vi "Write ITX (1D).vi"(0 "Commands":string, 5 "filename":path, 7 "Notes":string, 8 "Array name":string, 9 "1D Array":dbl[](array[numeric])) -> ()   [LabVIEW 2016, in "Data.ITX.lvclass"]
uses:
  Data.ITX.lvclass
  Data/Data.lvclass
panel:
  out "String":string
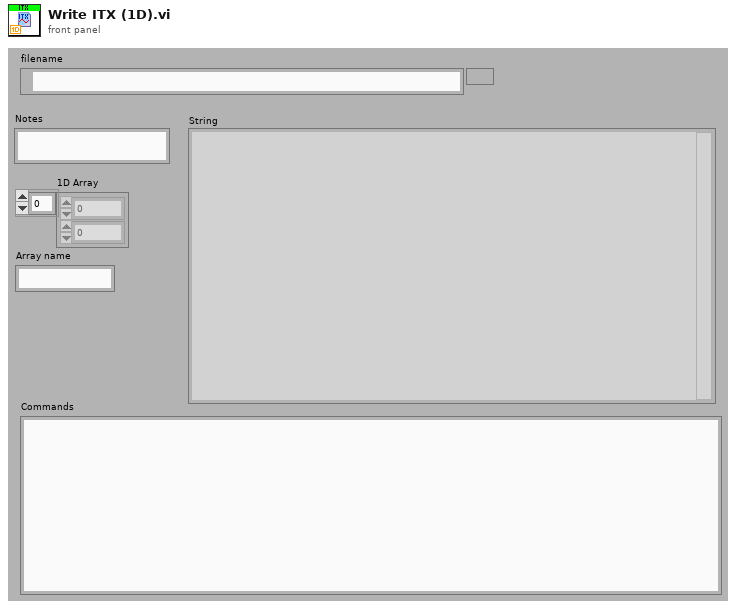
[diagram p1: front panel]
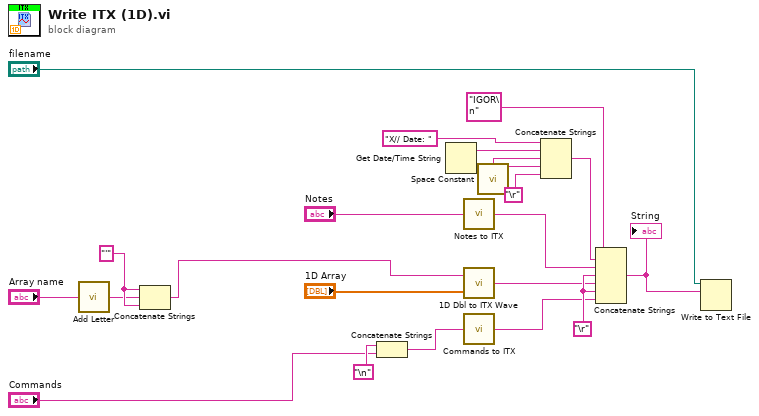
[diagram p0: block diagram]
diagram:
  w3 = "'" ("string")
  w17 = "\r"
  n1 = call "Add Letter.vi"("String"="Array name") -> ("output string"=w2:string)
  n2 = Concatenate Strings(w3, w2, w3) -> (w1:string)
  n3 = Concatenate Strings("\n", "Commands") -> (w8:string)
  n4 = Get Date/Time String() -> (date string=w21:string, time string=w22:string)  [unwired: 3 in]
  n5 = call "Notes to ITX.vi"("Notes"="Notes") -> ("ITX Notes"=w9:string)
  n6 = call "1D Dbl to ITX Wave.vi"("1D Array"="1D Array", "Wavename"=w1) -> ("ITX Wave"=w5:string)
  n7 = call "Commands to ITX.vi"("Commands"=w8) -> ("ITX Commands"=w7:string)
  n8 = call <vilib>:"Space Constant.vi"() -> ("String"=w15:string)
  n9 = Concatenate Strings("X// Date: " ("format string"), w21, w15, w22, "\r") -> (w20:string)
  n10 = Concatenate Strings("IGOR\n", w20, w9, w17, w5, w17, w7) -> (w16:string)
  "String" <- w16
  n11 = Write to Text File(file (use dialog)="filename", text=w16) -> ()  [unwired: 2 in, 3 out]
